vi "Humedad subVI.vi"() -> ()   [LabVIEW 2013]
panel:
  out "Numeric Indicator":dbl
  in  "Numeric Control":dbl
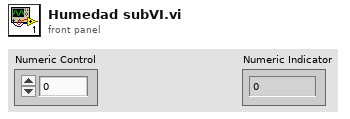
[diagram p1: front panel]
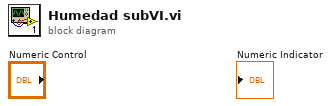
[diagram p0: block diagram]
diagram:
